vi "test_with_connector_pane.vi"(10 "Input 2":dbl, 11 "Input 1":dbl) -> (3 "Sum":dbl)   [LabVIEW 2026]
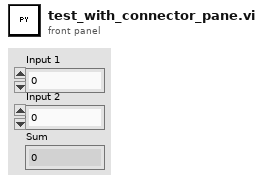
[diagram p1: front panel]
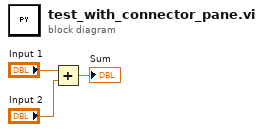
[diagram p0: block diagram]
diagram:
  n1 = Add(x="Input 1", y="Input 2") -> (x+y=→"Sum":dbl)
